vi "FPGA_X value calulate.vi"(9 "X Offset":i16, 10 "X Amplitude":fxp<+,16,0> format="%.16g", 11 "X Limited":i16) -> (3 "数值输入控件":i16)   [LabVIEW 2015]
uses:
  <vilib>/rvi/FXPMathLib/FxpMul/XNode/nifxpmath_Multiplier.xnode
  <vilib>/rvi/FXPMathLib/sim/FxpSim.dll
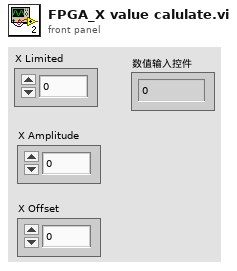
[diagram p1: front panel]
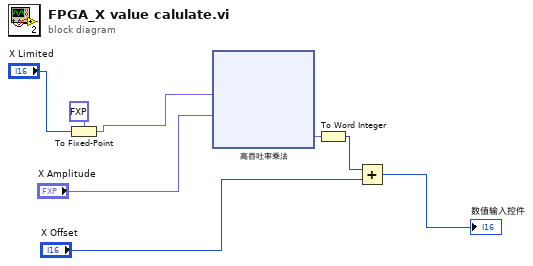
[diagram p0: block diagram]
diagram:
  n1 = To Fixed-Point(fixed-point type=fxp<+/-,17,17> 0.0 ("定点"), number="X Limited") -> (fixed-point=w2:fxp<+/-,17,17>)
  n2 = xnode ("高吞吐率乘法")("x"=w2, "y"="X Amplitude") -> ("x*y"=w5:fxp<+/-,16,16>)
  n3 = To Word Integer(number=w5) -> (16bit integer=w6:i16)
  n4 = Add(x=w6, y="X Offset") -> (x+y=→"数值输入控件":i16)
